vi "Configure Temperature Parameters.vi"(0 "VISA resource name":refnum<visa-resource-name>, 1 "Sensor (0: Thermocouple)":i32(ring) items=["Thermocouple", "Internal"], 2 "Reference Junction Type (0: Internal)":i32(ring) items=["Internal", "Simulated"], 5 "Simulated Reference Temp (23 C)":dbl=23.0, 7 "Thermocouple Type (0: J)":i32(ring) items=["J", "K", "T", "E", "R", "S", "B", "N"], 9 "Temperature Resolution (6)":i32=6, 11 "error in (no error)":errorcluster, 12 "Unit (0: Celsius)":i32(ring) items=["Celsius", "Fahrenheit", "Kelvin"]) -> (4 "VISA resource name out":refnum<visa-resource-name>, 15 "error out":errorcluster)   [LabVIEW 2011, in "Keithley 2182.lvlib"]
doc: "Configures the temperature measurements.\n\nThe Model 2182 has two temperature measurement functions: TEMP1 and TEMP2. TEMP1 is available for input Channel 1 and TEMP2 is available for Channel 2.\n\nDepending on which thermocouple type is used (J, K, T, E, R, S, B, or N), the Model 2182 can measure temperature from -200 deg. C to 1820 deg. C."
uses:
  Keithley 2182.lvlib
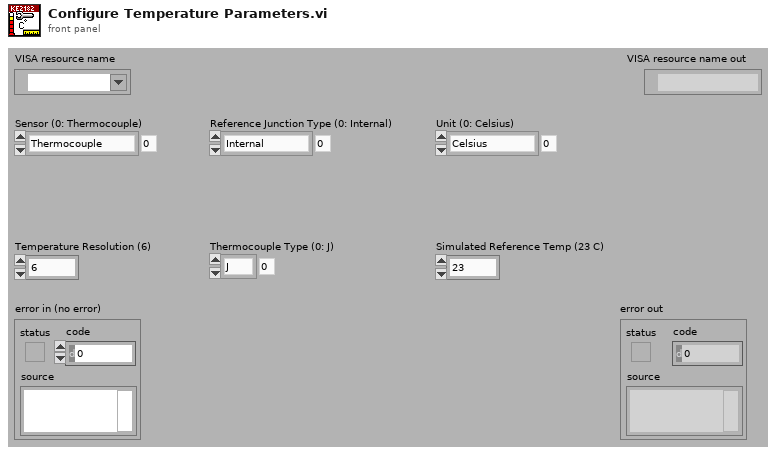
[diagram p1: front panel]
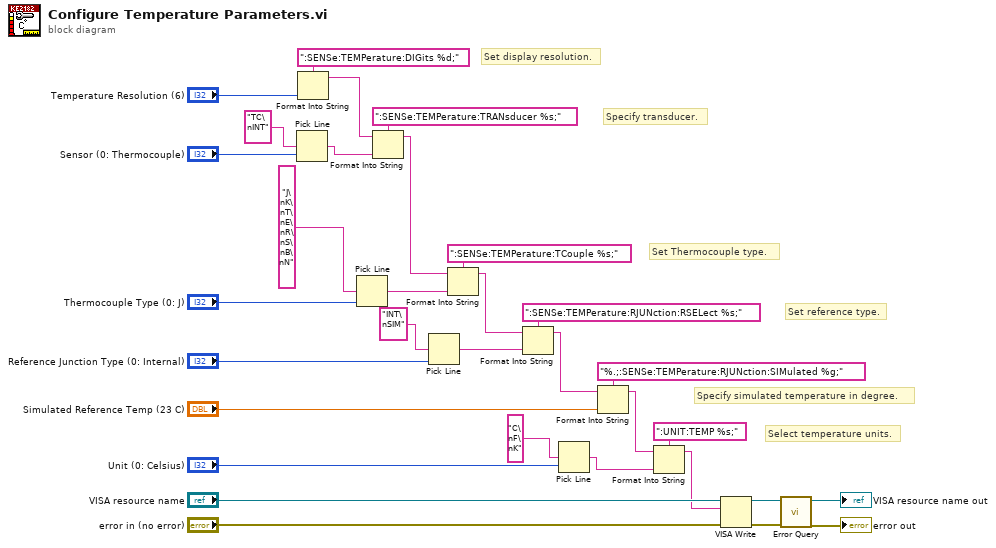
[diagram p0: block diagram]
diagram:
  # "Select temperature units."
  # "Specify simulated temperature in degree."
  # "Set reference type."
  # "Set Thermocouple type."
  # "Specify transducer."
  # "Set display resolution."
  n1 = Pick Line(multi-line string="TC\nINT", line index="Sensor (0: Thermocouple)") -> (output string=w15:string)  [unwired: 1 in]
  n2 = Format Into String(format string=":SENSe:TEMPerature:DIGits %d;", "Temperature Resolution (6)") -> (resulting string=w30:string)  [unwired: 2 in, 1 out]
  n3 = Pick Line(multi-line string="J\nK\nT\nE\nR\nS\nB\nN", line index="Thermocouple Type (0: J)") -> (output string=w4:string)  [unwired: 1 in]
  n4 = Format Into String(format string=":SENSe:TEMPerature:TRANsducer %s;", initial string=w30, w15) -> (resulting string=w28:string)  [unwired: 1 in, 1 out]
  n5 = Pick Line(multi-line string="INT\nSIM", line index="Reference Junction Type (0: Internal)") -> (output string=w2:string)  [unwired: 1 in]
  n6 = Format Into String(format string=":SENSe:TEMPerature:TCouple %s;", initial string=w28, w4) -> (resulting string=w26:string)  [unwired: 1 in, 1 out]
  n7 = Format Into String(format string=":SENSe:TEMPerature:RJUNction:RSELect %s;", initial string=w26, w2) -> (resulting string=w24:string)  [unwired: 1 in, 1 out]
  n8 = Pick Line(multi-line string="C\nF\nK", line index="Unit (0: Celsius)") -> (output string=w9:string)  [unwired: 1 in]
  n9 = Format Into String(format string="%.;:SENSe:TEMPerature:RJUNction:SIMulated %g;", initial string=w24, "Simulated Reference Temp (23 C)") -> (resulting string=w7:string)  [unwired: 1 in, 1 out]
  n10 = Format Into String(format string=":UNIT:TEMP %s;", initial string=w7, w9) -> (resulting string=w8:string)  [unwired: 1 in, 1 out]
  n11 = VISA Write(VISA resource name="VISA resource name", write buffer=w8, error in (no error)="error in (no error)") -> (VISA resource name out=w19:refnum<visa-resource-name>, error out=w18:errorcluster)  [unwired: 1 out]
  n12 = call "Error Query.vi"("error in (no error)"=w18, "VISA resource name"=w19) -> ("error out"=→"error out":errorcluster, "VISA resource name out"=→"VISA resource name out":refnum<visa-resource-name>)  [unwired: 6 in, 2 out]
